vi "Inheritance Example.vi"() -> ()   [LabVIEW 2019]
uses:
  Code/Shared/TCP Packet/packet type STYP.ctl
  Code/Shared/Map/Map.lvclass
  C:/projects/labview_multiplayer_snake/Main Codeline/Software/Code/Shared/TCP Packet/Packet.lvclass
  Code/Shared/Score/Score.lvclass
  Code/Shared/TCP Packet/Packet.lvclass
panel:
  out "Array 2":T1[](array[typedef])
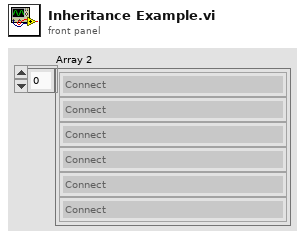
[diagram p1: front panel]
types:
  T1 = typedef "Packet.lvclass/packet type STYP.ctl" = enum16{"Connect", "Disconnect", "Direction", "Score", "Map"}
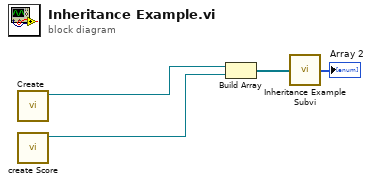
[diagram p0: block diagram]
diagram:
  n1 = call "Create.vi"() -> ("Map out"=w4:refnum<class "Map.lvclass">)  [unwired: 10 in, 1 out]
  n2 = call "create Score.vi"() -> ("Score out"=w3:refnum<class "Score.lvclass">)  [unwired: 10 in, 1 out]
  n3 = Build Array(w4, w3) -> (w2:refnum<class "Packet.lvclass">[])
  n4 = call "Inheritance Example Subvi.vi"("Array"=w2) -> ("Array 2"=→"Array 2":T1[])
